vi "Read RunVirtual.vi"(8 "error in (no error)":errorcluster, 11 "DriveTrain in":refnum<class "DriveTrain.lvclass">) -> (0 "error out":errorcluster, 2 "RunVirtual":bool, 3 "DriveTrain out":refnum<class "DriveTrain.lvclass">)   [LabVIEW 2013, in "DriveTrain.lvlib" / "DriveTrain.lvclass"]
uses:
  DriveTrain.lvclass
  DriveTrain.lvclass/DriveTrain.ctl
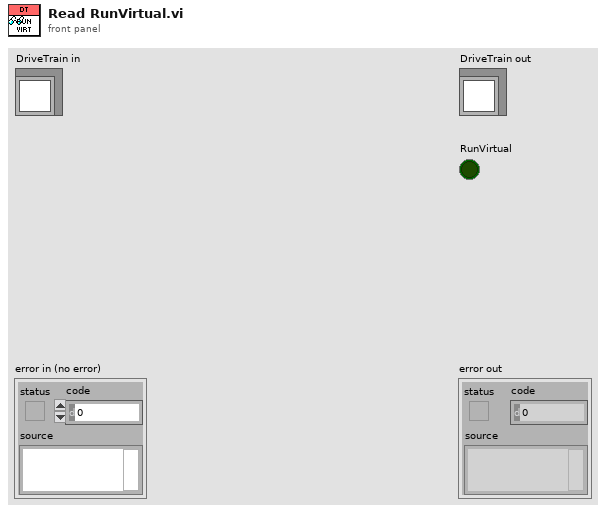
[diagram p1: front panel]
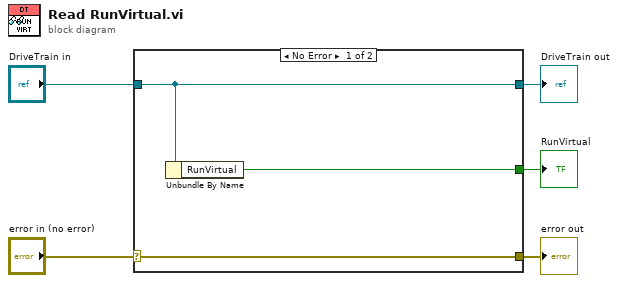
[diagram p0: block diagram]
diagram:
  n1 = case shown="No Error" "error in (no error)" {
    selector: "error in (no error)" -> [w8 w9]
    tunnel: [w8 w9] -> w4
    tunnel: [w7 w10] -> w2
    tunnel: "DriveTrain in" -> [w7 w10]
    tunnel: [w6 _] -> w1
    frame No Error {
      n2 = Unbundle By Name(w7) -> ("RunVirtual"=w6:bool)
    }
    frame Error {
    }
  }
  "error out" <- w4
  "DriveTrain out" <- w2
  "RunVirtual" <- w1
